vi "Write Static Position.vi"(8 "error in (no error)":errorcluster, 10 "Static Position":T1, 11 "Static Overlay in":refnum<class "Static Overlay.lvclass">) -> (0 "error out":errorcluster, 3 "Static Overlay out":refnum<class "Static Overlay.lvclass">)   [LabVIEW 2014, in "Static Overlay.lvclass"]
uses:
  Static Overlay.lvclass
  Static Position.ctl
  Static Overlay.lvclass/Static Overlay.ctl
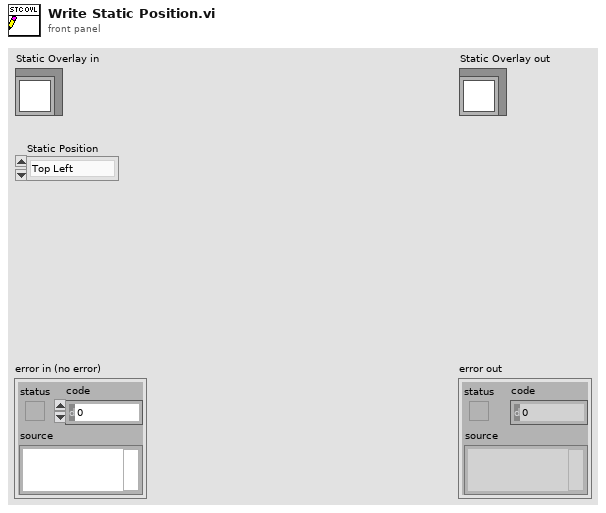
[diagram p1: front panel]
types:
  T1 = typedef "Static Overlay.lvclass/Static Position.ctl" = enum16{"Top Left", "Top Center", "Top Right", "Center", "Bottom Left", "Bottom Center", "Bottom Right"}
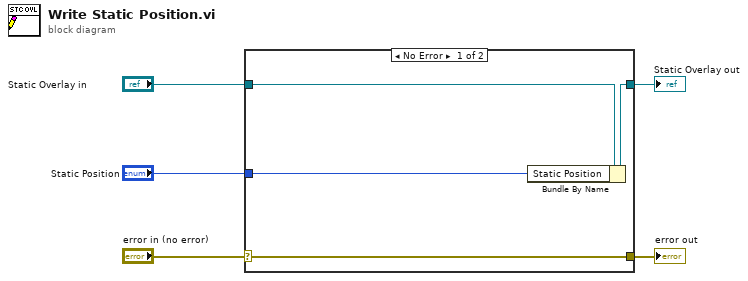
[diagram p0: block diagram]
diagram:
  n1 = case shown="No Error" "error in (no error)" {
    selector: "error in (no error)" -> [w9 w10]
    tunnel: [w9 w10] -> w4
    tunnel: [w7 w11] -> w2
    tunnel: "Static Overlay in" -> [w8 w11]
    tunnel: "Static Position" -> [w6 _]
    frame No Error {
      n2 = Bundle By Name(cluster=w8, "Static Position"=w6) -> (w7:refnum<class "Static Overlay.lvclass">)
    }
    frame Error {
    }
  }
  "error out" <- w4
  "Static Overlay out" <- w2
